vi "AddCredit.vi"(8 "error in (no error)":errorcluster, 10 "Coins Cluster":T1, 11 "Coins in":refnum<class "Coins.lvclass">) -> (0 "error out":errorcluster, 3 "Coins out":refnum<class "Coins.lvclass">)   [LabVIEW 2020, in "Coins.lvlib" / "Coins.lvclass"]
uses:
  Coins.lvclass
  C:/Program Files (x86)/National Instruments/LabVIEW 2020/vi.lib/ActorFramework/Actor/Actor.lvclass
  <vilib>/ActorFramework/Actor/Actor.lvclass/Actor.ctl
  Coins.lvclass/Coins.ctl
  UI Actor Messages/AddCredit Msg/AddCredit Msg.lvclass/AddCredit Msg.ctl
  <vilib>/ActorFramework/Message Enqueuer/Message Enqueuer.lvclass/Message Enqueuer.ctl
  <vilib>/ActorFramework/Message Enqueuer/Enqueue.vi
  UI Actor Messages/AddCredit Msg/AddCredit Msg.lvclass
  C:/Program Files (x86)/National Instruments/LabVIEW 2020/vi.lib/ActorFramework/Message/Message.lvclass
  <vilib>/ActorFramework/Message Priority Queue/Priority Enqueue.vi
  <vilib>/ActorFramework/Actor/Actor.lvclass
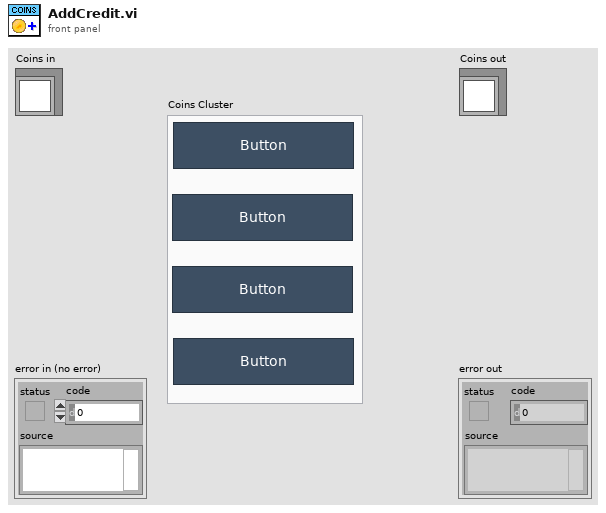
[diagram p1: front panel]
types:
  T1 = cluster{"Coin 1":bool, "Coin 2":bool, "Coin 3":bool, "Coin 4":bool}
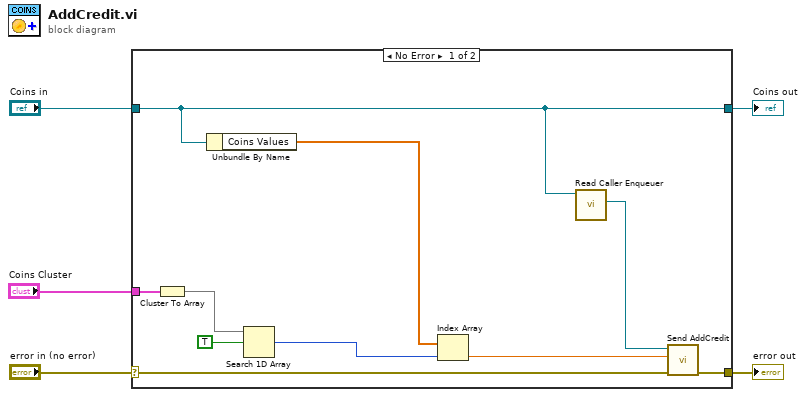
[diagram p0: block diagram]
diagram:
  n1 = case shown="No Error" "error in (no error)" {
    selector: "error in (no error)" -> [w15 w17]
    tunnel: [w14 w17] -> w4
    tunnel: [w12 w16] -> w2
    tunnel: "Coins in" -> [w12 w16]
    tunnel: "Coins Cluster" -> [w9 _]
    frame No Error {
      n2 = Cluster To Array(cluster=w9) -> (array=w8:bool[])
      n3 = Unbundle By Name(w12) -> ("Coins Values"=w11:dbl[])
      n4 = Search 1D Array(1D array=w8, element=TRUE) -> (index of element=w6:i32)  [unwired: 1 in]
      n5 = Index Array(array=w11, index=w6) -> (element=w10:dbl)
      n6 = call <vilib>:"Read Caller Enqueuer.vi"("Actor"=w12) -> ("Caller Enqueuer"=w13:refnum<class "Message Enqueuer.lvclass">)  [unwired: 10 in]
      n7 = call "Send AddCredit.vi"("error in (no error)"=w15, "Credit Added"=w10, "Message Enqueuer"=w13) -> ("error out"=w14:errorcluster)  [unwired: 7 in, 1 out]
    }
    frame Error {
    }
  }
  "error out" <- w4
  "Coins out" <- w2
